vi "3.1.1.1-VectorNav Read Write.vi"() -> ()   [LabVIEW 2010]
panel:
  out "Boolean 2":bool
  out "Boolean":bool
  out "Yaw":dbl
  out "Reply":string
  in  "Command":string="$VNRRG,08*7B"
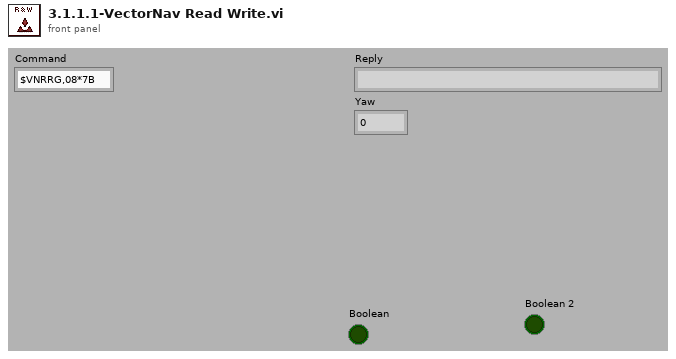
[diagram p1: front panel]
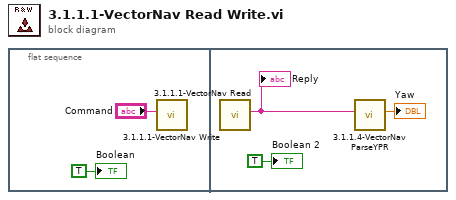
[diagram p0: block diagram]
diagram:
  n1 = flat-sequence {
    frame #0 {
      n2 = call "3.1.1.1-VectorNav Write.vi"("Command"="Command") -> ()  [unwired: 11 in]
      "Boolean" <- TRUE ("Boolean")
    }
    frame #1 {
      n3 = call "3.1.1.1-VectorNav Read.vi"() -> ("Reply"=w5:string)  [unwired: 11 in]
      "Reply" <- w5
      n4 = call "3.1.1.4-VectorNav ParseYPR.vi"("Input String"=w5) -> ("Yaw"=→"Yaw":dbl)  [unwired: 8 in, 2 out]
      "Boolean 2" <- TRUE ("Boolean")
    }
  }
